vi "PH_Beckhoff-16BB.open PSDB Connection.vi"(0 "i ref in":refnum<vi>, 5 "error in":errorcluster) -> (14 "i ref out":refnum<vi>, 19 "error out":errorcluster)   [LabVIEW 2014, in "PH_Beckhoff-16BB.lvlib"]
doc: "This VI opens the connection to the PSDB to get the necessary IDs and opens the related DIM services."
uses:
  PH_Beckhoff-16BB.lvlib
  PH_Basics/PH_PSDBWriter/PH_PSDBWriter.PHELIX-Subsystems.ctl
  PH_Beckhoff_Common/PH_Beckhoff_Common.former PSDB classes.ctl
  PH_Basics/PH_PSDBWriter/PH_PSDBWriter.Data Status.ctl
  PH_Basics/PH_PSDBWriter/PH_PSDBWriter.lvlib
  CSlibraries-extern/DimLVEvent/LVDimInterface/LVDimInterface.lvlib
  PH_Beckhoff_Common/PH_Beckhoff_Common.lvlib
  PH_Basics/PH_Common/PH_Common.lvlib
panel:
  in  "PHELIX Subsysteme":T1 items=["Miscellaneous", "fs-Frontend", "ns-Frontend", "PreAmp", "MainAmp", "MAS", "COS", "Beamline", "Experiment Laserbay", "Experiment Laserlabor", "Experiment Z6", "Timing", "Pulsed Power"]
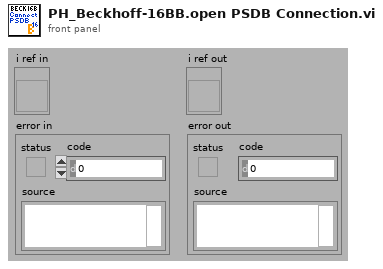
[diagram p1: front panel]
types:
  T1 = typedef "PH_PSDBWriter.lvlib/PH_PSDBWriter.PHELIX-Subsystems.ctl" = i32
  T2 = typedef "PH_Beckhoff_Common.lvlib/PH_Beckhoff_Common.former PSDB classes.ctl" = enum16{"PP Conductivity", "PP Mercury", "PA Chiller"}
  T3 = typedef "PH_Beckhoff-16BB.lvlib/PH_Beckhoff-16BB.i attribute.ctl" = cluster{"PA Chiller":cluster{"PSDB":cluster{"Status Service ID":i32, "Instance ID":i32, "Data Status":T4, "Ref Status":refnum<vi>, "Error Code":i32}, "Status":cluster{"GUI Ref":refnum<vi>, "Status Service ID":i32, "Status":T5}, "DIs":cluster{"Flow Control":cluster{"GUI Ref":refnum<vi>, "# in Data":i32}, "High-Temp":cluster{"GUI Ref":refnum<vi>, "# in Data":i32}, "Conductivity":cluster{"GUI Ref":refnum<vi>, "# in Data":i32}, "Niveau":cluster{"GUI Ref":refnum<vi>, "# in Data":i32}}, "PSDB Thread":cluster{"Ref":refnum<vi>, "Q-Ref":refnum<queue>}}, "PSDB":cluster{"Shot #":i32, "Subsystem":T1}, "Racktype":string, "PSDB Credentials":T6}
  T4 = typedef "PH_PSDBWriter.lvlib/PH_PSDBWriter.Data Status.ctl" = i16
  T5 = typedef "PH_StatusHandler.lvlib/PH_StatusHandler.Status.ctl" = i16
  T6 = typedef "PH_Common.lvlib/PH_Connection.PSDB Credentials.ctl" = cluster{"PW":string, "ID":string, "DS":string}
  T7 = cluster{"Instancename":string, "Classname":string}
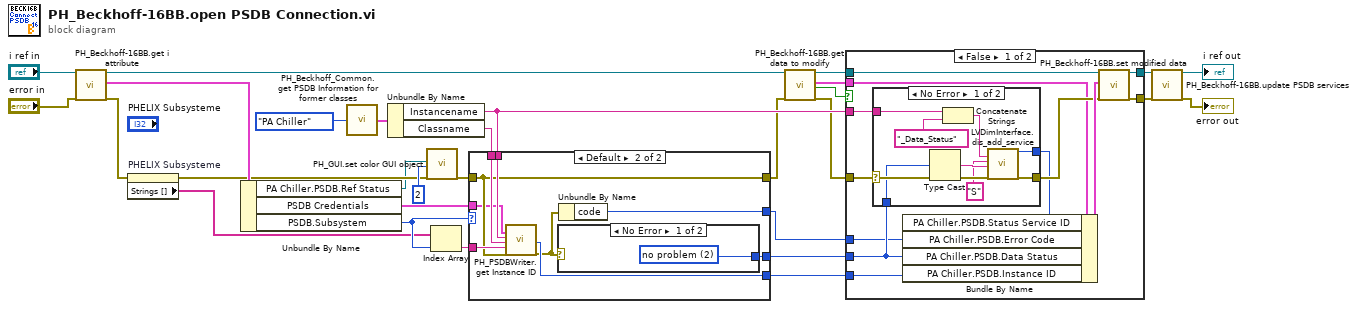
[diagram p0: block diagram]
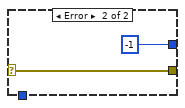
[diagram p2: hidden frame]
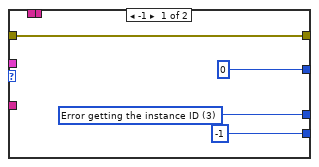
[diagram p4: hidden frame]
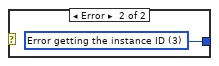
[diagram p5: hidden frame]
diagram:
  n1 = call "PH_Beckhoff-16BB.get i attribute.vi"("i ref in"="i ref in", "error in (no error)"="error in") -> ("i ref out"=w28:refnum<vi>, "i attribute"=w29:T3, "error out"=w26:errorcluster)  [unwired: 15 in]
  n2 = property on="PHELIX Subsysteme" class="Ring (strict)"(error in=w26) -> (error out=w8:errorcluster, "Strings []"=w10:string[])  [unwired: 1 in, 1 out]
  n3 = Unbundle By Name(w29) -> ("PA Chiller.PSDB.Ref Status"=w6:refnum<vi>, "PSDB Credentials"=w1:T6, "PSDB.Subsystem"=w23:T1)
  n4 = call "PH_Beckhoff_Common.get PSDB Information for former classes.vi"("PSDB Classes"=PH_Beckhoff_Common.former_PSDB_classes."PA Chiller") -> ("PSDB Information"=w22:T7)
  n5 = Unbundle By Name(w22) -> ("Instancename"=w20:string, "Classname"=w19:string)
  n6 = call "PH_GUI.set color GUI object.vi"("GUI object Ref"=w6, "State"=2, "error in (no error)"=w8) -> ("error out"=w7:errorcluster)  [unwired: 16 in]
  n7 = Index Array(array=w10, index=w23) -> (element=w24:string)
  n8 = case shown="Default" w23 {
    tunnel: [w33 w42] -> w18
    tunnel: [-1 ("instance_id") w37] -> w17
    tunnel: w7 -> [w31 w35]
    tunnel: [w31 w35] -> w12
    tunnel: [0 ("code") w41] -> w16
    tunnel: w24 -> [_ w38]
    tunnel: w20 -> [_ w40]
    tunnel: w19 -> [_ w39]
    tunnel: w1 -> [_ w34]
    frame -1 {
      w33 = T4 3 items=["no info", "no Data collection", "no problem", "Error getting the instance ID", "Error writing Data to data base", "Error concerning the subsystem"] ("Metadata.Data Status")
    }
    frame Default {
      n9 = call "PH_PSDBWriter.get Instance ID.vi"("PSDB Credentials"=w34, "Instace Name"=w40, "Class"=w39, "Subsystem"=w38, "error in"=w35) -> ("instance_id"=w37:i32, "error out"=w36:errorcluster)  [unwired: 13 in]
      n10 = case shown="No Error" w36 {
        tunnel: [w43 w44] -> w42
        frame No Error {
          w43 = T4 2 items=["no info", "no Data collection", "no problem", "Error getting the instance ID", "Error writing Data to data base"] ("Metadata.Data Status")
        }
        frame Error {
          w44 = T4 3 items=["no info", "no Data collection", "no problem", "Error getting the instance ID", "Error writing Data to data base"] ("Metadata.Data Status")
        }
      }
      n11 = Unbundle By Name(w36) -> ("code"=w41:i32)
    }
  }
  n12 = call "PH_Beckhoff-16BB.get data to modify.vi"("i ref in"=w28, "error in (no error)"=w12) -> ("i ref out"=w14:refnum<vi>, "i attribute"=w15:T3, "timed out"=w11:bool, "error out"=w13:errorcluster)  [unwired: 14 in]
  n13 = case shown="False" w11 {
    tunnel: [w56 w69] -> w4
    tunnel: [w55 w68] -> w2
    tunnel: w20 -> [w52 _]
    tunnel: w18 -> [w50 _]
    tunnel: w17 -> [w49 _]
    tunnel: w16 -> [w48 _]
    tunnel: w15 -> [w47 _]
    tunnel: w14 -> [w46 w69]
    tunnel: w13 -> [w45 w68]
    frame False {
      n14 = case shown="No Error" w45 {
        selector: w45 -> [w63 w67]
        tunnel: [w65 -1 ("my_serviceID")] -> w51
        tunnel: [w64 w67] -> w53
        tunnel: w52 -> [w58 _]
        tunnel: w50 -> [w57 _]
        frame No Error {
          n15 = Type Cast(x=w57) -> (*(type *) &x=w62:string)  [unwired: 1 in]
          n16 = Concatenate Strings(w58, "_Data_Status" ("string")) -> (w60:string)
          n17 = call "LVDimInterface.dis_add_service.vi"("serviceName"=w60, "typeDescriptor"="S", "data"=w62, "error in (no error)"=w63) -> ("my_serviceID"=w65:i32, "error out"=w64:errorcluster)  [unwired: 14 in]
        }
        frame Error {
        }
      }
      n18 = Bundle By Name(cluster=w47, "PA Chiller.PSDB.Status Service ID"=w51, "PA Chiller.PSDB.Error Code"=w48, "PA Chiller.PSDB.Data Status"=w50, "PA Chiller.PSDB.Instance ID"=w49) -> (w54:T3)
      n19 = call "PH_Beckhoff-16BB.set modified data.vi"("i ref in"=w46, "i attribute"=w54, "error in (no error)"=w53) -> ("i ref out"=w56:refnum<vi>, "error out"=w55:errorcluster)  [unwired: 15 in]
    }
    frame True {
    }
  }
  n20 = call "PH_Beckhoff-16BB.update PSDB services.vi"("i ref in"=w4, "error in"=w2) -> ("i ref out"=→"i ref out":refnum<vi>, "error out"=→"error out":errorcluster)  [unwired: 16 in]
